vi "GoToBall.vi"(8 "error in (no error)":errorcluster, 9 "Ball":refnum<class "Ball.lvclass">, 10 "Robot":refnum<class "Robot.lvclass">, 11 "GoToSkill in":refnum<class "GoToSkill.lvclass">) -> (0 "error out":errorcluster, 2 "Robot out":refnum<class "Robot.lvclass">, 3 "GoToSkill out":refnum<class "GoToSkill.lvclass">)   [LabVIEW 2023, in "GoToSkill.lvclass"]
uses:
  GoToSkill.lvclass
  Ball_class/Ball.lvclass
  C:/Users/ebert/Documents/codes/SSL/repo/SSL_AI/Object_class/Object.lvclass
  Robot_class/Robot.lvclass
  Object_class/Object.lvclass/Object.ctl
  Object_class/Read position(x,y).vi
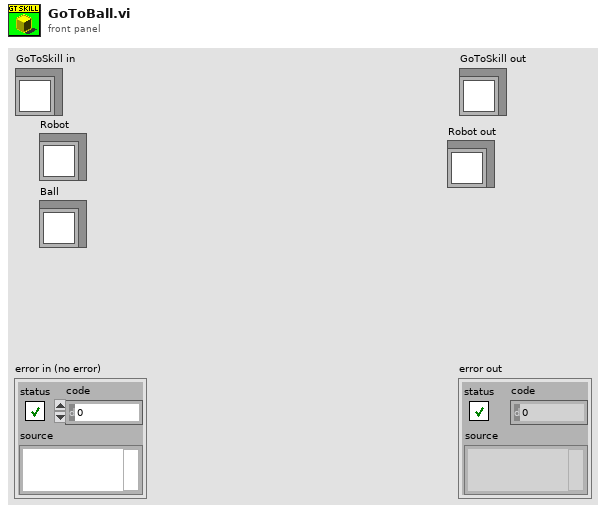
[diagram p1: front panel]
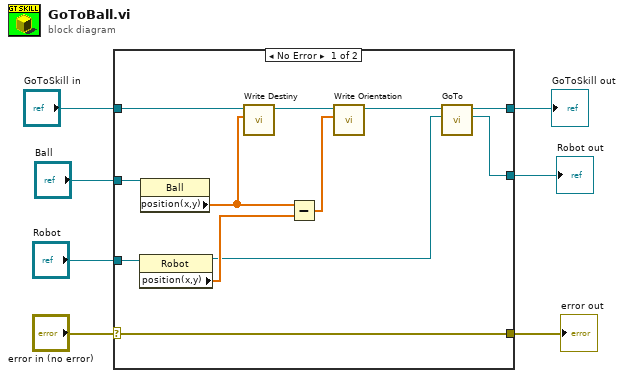
[diagram p0: block diagram]
diagram:
  n1 = case shown="No Error" "error in (no error)" {
    selector: "error in (no error)" -> [w19 w22]
    tunnel: [w19 w22] -> w6
    tunnel: [w9 w21] -> w4
    tunnel: "GoToSkill in" -> [w17 w21]
    tunnel: "Ball" -> [w18 _]
    tunnel: "Robot" -> [w16 w20]
    tunnel: [w8 w20] -> w1
    frame No Error {
      n2 = property class="Robot"(reference=w16) -> (reference out=w11:refnum<class "Robot.lvclass">, "position(x,y)"=w14:dbl[])  [unwired: 1 in, 1 out]
      n3 = property class="Ball"(reference=w18) -> ("position(x,y)"=w15:dbl[])  [unwired: 1 in, 2 out]
      n4 = call-dynamic "Write Destiny.vi"("Destiny"=w15, "GoToSkill in"=w17) -> ("GoToSkill out"=w12:refnum<class "GoToSkill.lvclass">)  [unwired: 8 in, 1 out]
      n5 = Subtract(x=w15, y=w14) -> (x-y=w13:dbl[])
      n6 = call-dynamic "Write Orientation.vi"("Orientation"=w13, "GoToSkill in"=w12) -> ("GoToSkill out"=w10:refnum<class "GoToSkill.lvclass">)  [unwired: 8 in, 1 out]
      n7 = call-dynamic "GoTo.vi"("Robot"=w11, "GoToSkill in"=w10) -> ("Robot out"=w8:refnum<class "Robot.lvclass">, "GoToSkill out"=w9:refnum<class "GoToSkill.lvclass">)  [unwired: 7 in, 1 out]
    }
    frame Error {
    }
  }
  "error out" <- w6
  "GoToSkill out" <- w4
  "Robot out" <- w1
